vi "rszvl Configure Spectrogram Sweep.vi"(8 "error in (no error)":errorcluster, 9 "Continuous (On)":bool=TRUE, 11 "VISA resource name":refnum<visa-resource-name>) -> (0 "error out":errorcluster, 3 "VISA resource name out":refnum<visa-resource-name>)   [LabVIEW 2014]
doc: "This VI starts a continuous sweep measurement or stops it and switches to single sweep mode.\n\nNote: \n\n(1) This VI is available only with option R&S FS-K14.\n\nAttribute(s):\nRSZVL_ATTR_SWEEP_MODE_CONTINUOUS\n\nRemote-control command(s):\nINITiate<1|2>:CONTinuous OFF | ON"
uses:
  Instance           1 41Saved   rszvl Configure Spectrogram Sweep .vi
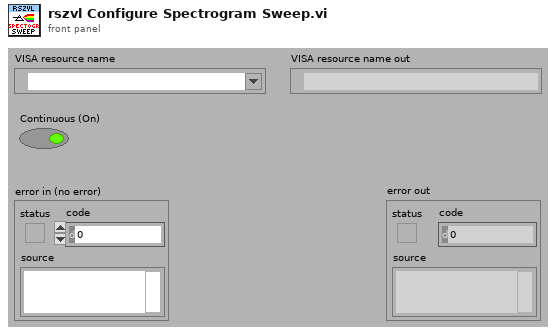
[diagram p1: front panel]
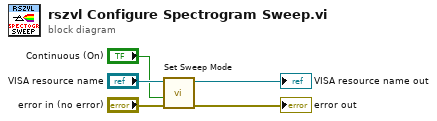
[diagram p0: block diagram]
diagram:
  n1 = call "Set Sweep Mode"("error in (no error)"="error in (no error)", "Sweep Mode (OFF)"="Continuous (On)", "instrument handle"="VISA resource name") -> ("error out"=→"error out":errorcluster, "instrument handle out"=→"VISA resource name out":refnum<visa-resource-name>)  [unwired: 7 in]
